vi "GetType.vi"(8 "error in (no error)":errorcluster, 11 "AbortAllMovements Msg":refnum<class "AbortAllMovements Msg.lvclass">) -> (0 "error out":errorcluster, 2 "Data Sample":variant, 3 "AbortAllMovements Msg":refnum<class "AbortAllMovements Msg.lvclass">)   [LabVIEW 2016, in "CS++Motor.lvlib" / "AbortAllMovements Msg.lvclass"]
uses:
  AbortAllMovements Msg.lvclass
  AbortAllMovements Msg.lvclass/AbortAllMovements Msg.ctl
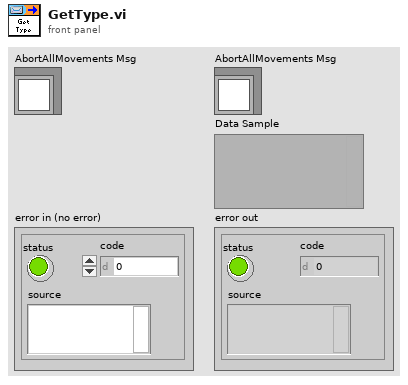
[diagram p1: front panel]
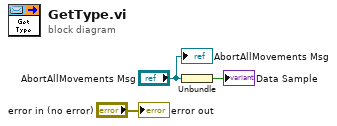
[diagram p0: block diagram]
diagram:
  n1 = Unbundle("AbortAllMovements Msg") -> (→"Data Sample":bool)
  "error out" <- "error in (no error)"
  "AbortAllMovements Msg" <- "AbortAllMovements Msg"
